vi "Entry.vi"(8 "error in (no error)":errorcluster, 11 "New State":refnum<class "Finishing Command.lvclass">) -> (0 "error out":errorcluster, 3 "State out":refnum<class "Finishing Command.lvclass">)   [LabVIEW 2014, in "Robot Actor Framework.lvlib" / "Command Processor Actor.lvlib" / "Finishing Command.lvclass"]
doc: "This is an abstract method. Override this method to define the behavior when you enter the state."
uses:
  Finishing Command.lvclass
  Command Processor Actor Class/Command Processor States.ctl
  <vilib>/ActorFramework/Message Enqueuer/Message Enqueuer.lvclass/Message Enqueuer.ctl
  <vilib>/ActorFramework/Message Enqueuer/Enqueue.vi
  <vilib>/ActorFramework/Message Priority Queue/Priority Enqueue.vi
  <vilib>/ActorFramework/Stop Msg/Stop Msg.lvclass
  Command Processor Actor Class/Command Processor Actor.lvclass
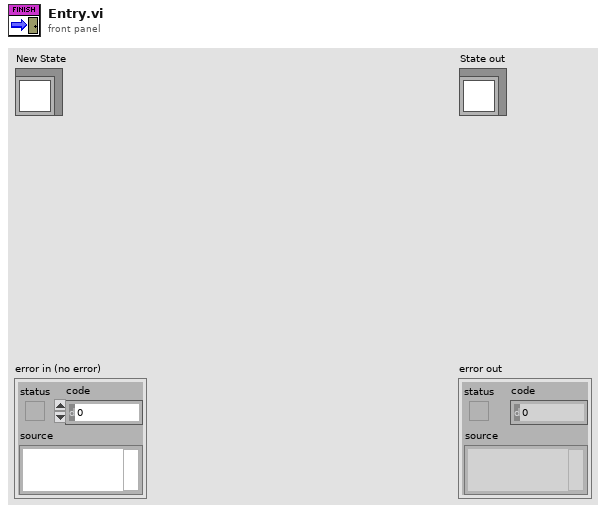
[diagram p1: front panel]
types:
  T1 = typedef "Robot Actor Framework.lvlib/Command Processor Actor.lvlib/Command Processor Actor.lvclass/Command Processor States.ctl" = enum16{"Unknown", "No Command", "Running Command", "Starting Command", "Stopping Command", "Finishing Command"}
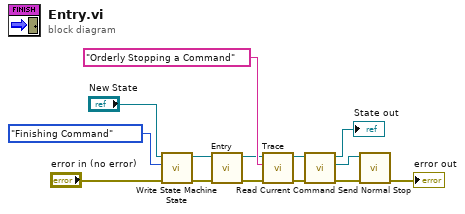
[diagram p0: block diagram]
diagram:
  n1 = call-dynamic "Write State Machine State.vi"("error in (no error)"="error in (no error)", "Command Processor State"=Command_Processor_States."Finishing Command", "Command Processor Actor in"="New State") -> ("error out"=w5:errorcluster, "Command Processor Actor out"=w6:refnum<class "Finishing Command.lvclass">)  [unwired: 7 in]
  n2 = call-parent "Entry.vi"("error in (no error)"=w5, "New State"=w6) -> ("error out"=w4:errorcluster, "State out"=w3:refnum<class "Finishing Command.lvclass">)  [unwired: 8 in]
  n3 = call-dynamic "Trace.vi"("error in (no error)"=w4, "Command Processor Action"="Orderly Stopping a Command", "Command Processor Actor in"=w3) -> ("error out"=w11:errorcluster, "Command Processor Actor out"=w8:refnum<class "Finishing Command.lvclass">)  [unwired: 7 in]
  n4 = call-dynamic "Read Current Command.vi"("error in (no error)"=w11, "Command Processor in"=w8) -> ("error out"=w10:errorcluster, "Actor Framework:Message Enqueuer"=w9:refnum<class "Message Enqueuer.lvclass">, "Command Processor out"=→"State out":refnum<class "Finishing Command.lvclass">)  [unwired: 7 in]
  n5 = call <vilib>:"Send Normal Stop.vi"("error in (no error)"=w10, "Message Enqueuer"=w9) -> ("error out"=→"error out":errorcluster)  [unwired: 9 in]
